vi "Processing_Tracks_Without_Problems-7.vi"(5 "[IN] Min TRK L":i32, 6 "[IN] Max angle between \ntwo displacements":dbl min=1.0 max=90.0 step=1.0, 7 "[IN] % linearity":i32, 8 "error IN":errorcluster, 9 "[IN] Movie Values":T2 {"Particle Fil Setups"."Type of particle filter"."Measurement Parameter" items=["Center of Mass X", "Center of Mass Y", "First Pixel X", "First Pixel Y", "Bounding Rect Left", "Bounding Rect Top", "Bounding Rect Right", "Bounding Rect Bottom", "Max Feret Diameter Start X", "Max Feret Diameter Start Y", "Max Feret Diameter End X", "Max Feret Diameter End Y", "Max Horiz. Segment Length Left", "Max Horiz. Segment Length Right", "Max Horiz. Segment Length Row", "-", "Bounding Rect Width", "Bounding Rect Height", "Bounding Rect Diagonal", "Perimeter", "Convex Hull Perimeter", "Holes' Perimeter", "Max Feret Diameter", "Equivalent Ellipse Major Axis", "Equivalent Ellipse Minor Axis", "Equivalent Ellipse Minor Axis (Feret)", "Equivalent Rect Long Side", "Equivalent Rect Short Side", "Equivalent Rect Diagonal", "Equivalent Rect Short Side (Feret)", "Average Horiz. Segment Length", "Average Vert. Segment Length", "Hydraulic Radius", "Waddel Disk Diameter", "-", "Area", "Holes' Area", "Particle & Holes' Area", "Convex Hull Area", "Image Area", "-", "Number of Holes", "Number of Horiz. Segments", "Number of Vert. Segments", "-", "Orientation", "Max Feret Diameter Orientation", "-", "% Area/Image Area", "% Area/(Particle & Holes' Area)", "Ratio of Equivalent Ellipse Axes", "Ratio of Equivalent Rect Sides", "-", "Elongation Factor", "Compactness Factor", "Heywood Circularity Factor", "Type Factor", "-", "Sum X", "Sum Y", "Sum XX", "Sum XY", "Sum YY", "Sum XXX", "Sum XXY", "Sum XYY", "Sum YYY", "-", "Moment of Inertia XX", "Moment of Inertia XY", "Moment of Inertia YY", "Moment of Inertia XXX", "Moment of Inertia XXY", "Moment of Inertia XYY", "Moment of Inertia YYY", "Norm. Moment of Inertia XX", "Norm. Moment of Inertia XY", "Norm. Moment of Inertia YY", "Norm. Moment of Inertia XXX", "Norm. Moment of Inertia XXY", "Norm. Moment of Inertia XYY", "Norm. Moment of Inertia YYY", "Hu Moment 1", "Hu Moment 2", "Hu Moment 3", "Hu Moment 4", "Hu Moment 5", "Hu Moment 6", "Hu Moment 7"]}, 11 "[IN] Tracks w/t Problems":T3(array[cluster])) -> (0 "error OUT":errorcluster, 2 "[OUT] Filtered Tracks":T3(array[cluster]), 3 "[OUT] Frame-to-Frame Displacements\n Extract From Tracks":dbl[][](array[numeric]))   [LabVIEW 2013]
doc: "SubVI processes the track depending on few parameters: linearity (processivity), length, area differences between connected particles (utilized the properties of the distribution of these differences)"
panel:
  out "[OUT] Filtered out\nShort Tracks":cluster{"Short Tracks":dbl[], "Start Pos":i32}[](array[cluster])
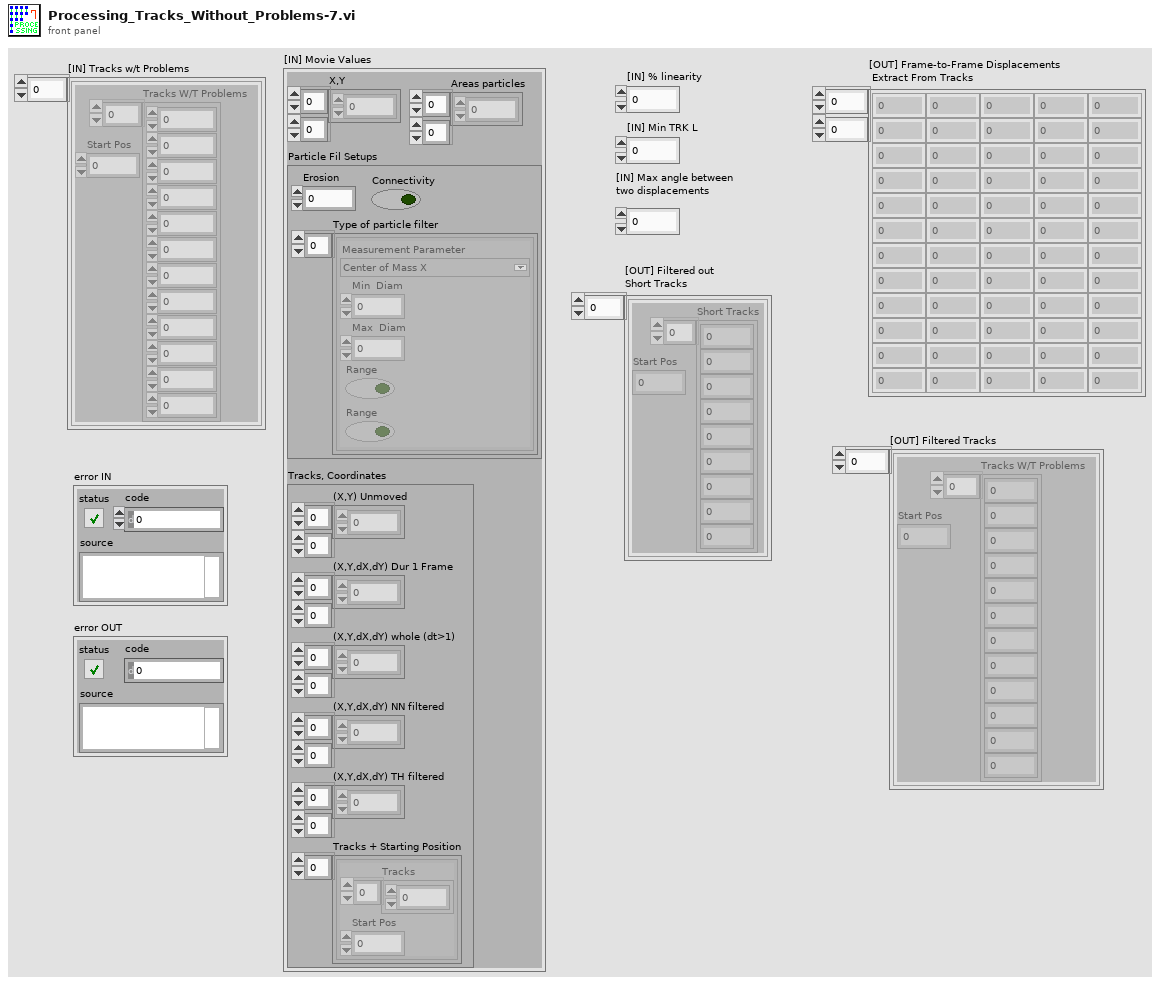
[diagram p1: front panel]
types:
  T1 = typedef "Particle Parameters" = i32
  T2 = cluster{"X,Y":dbl[][], "Areas particles":dbl[][], "Particle Fil Setups":cluster{"Erosion":i32, "Connectivity ":bool, "Type of particle filter":cluster{"Measurement Parameter":T1, "Min  Diam":dbl, "Max  Diam":dbl, "Range":bool, "Range":bool}[]}, "Tracks, Coordinates":cluster{"(X,Y) Unmoved":dbl[][], "(X,Y,dX,dY) Dur 1 Frame":dbl[][], "(X,Y,dX,dY) whole (dt>1)":dbl[][], "(X,Y,dX,dY) NN filtered":dbl[][], "(X,Y,dX,dY) TH filtered":dbl[][], "Tracks + Starting Position":cluster{"Tracks":dbl[], "Start Pos":i32}[]}}
  T3 = cluster{"Tracks W/T Problems":dbl[], "Start Pos":i32}[]
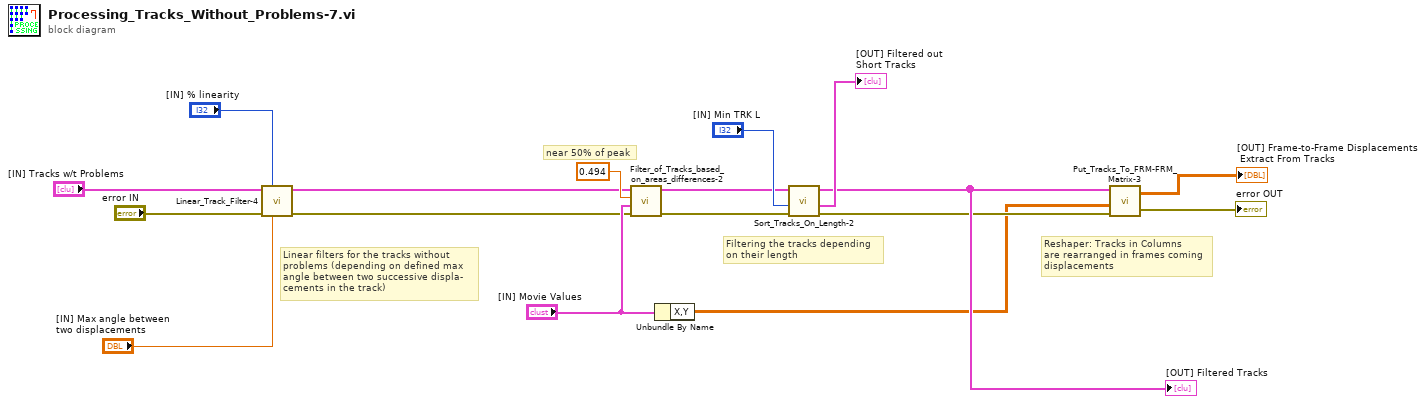
[diagram p0: block diagram]
diagram:
  # "near 50% of peak"
  # "Filtering the tracks depending\non their length"
  # "Linear filters for the tracks without \nproblems (depending on defined max\nangle between two successive displa-\ncements in the track)"
  # "Reshaper: Tracks in Columns\nare rearranged in frames coming\ndisplacements"
  n1 = call "Linear_Track_Filter-4.vi"("[IN] Max angle"="[IN] Max angle between \ntwo displacements", "[IN] % track linearity"="[IN] % linearity", "error IN"="error IN", "[IN] Tracks w/t Problems"="[IN] Tracks w/t Problems") -> ("error OUT"=w2:errorcluster, "[OUT] Linear Tracks (Filtered)"=w4:T3)  [unwired: 5 in, 1 out]
  n2 = call "Filter_of_Tracks_based_on_areas_differences-2.vi"("error IN"=w2, "[IN] Movie Values"="[IN] Movie Values", "[IN] Part of mean value (amplitude)\nFor making filtering criteria"=0.494 ("[IN] Part of mean value (amplitude)\nFor making filtering criteria"), "[IN] Tracks w/t Problems"=w4) -> ("error OUT"=w9:errorcluster, "[OUT] Stable Tracks (Filtered)"=w10:T3)  [unwired: 1 in, 1 out]
  n3 = Unbundle By Name("[IN] Movie Values") -> ("X,Y"=w7:dbl[][])
  n4 = call "Sort_Tracks_On_Length-2.vi"("error IN"=w9, "[IN] Min Track Length"="[IN] Min TRK L", "[IN] Tracks w/t Problems"=w10) -> ("error OUT"=w12:errorcluster, "[OUT] Short Tracks"=→"[OUT] Filtered out\nShort Tracks":cluster{"Short Tracks":dbl[], "Start Pos":i32}[], "[OUT] Long Tracks (Filtered)"=w13:T3)  [unwired: 2 in]
  "[OUT] Filtered Tracks" <- w13
  n5 = call "Put_Tracks_To_FRM-FRM_Matrix-3.vi"("error IN"=w12, "[IN] Matrix for Estimation \nSizes of Frame-to-Frame \nDisplacements from Tracks"=w7, "[IN] Tracks w/t Problems"=w13) -> ("error OUT"=→"error OUT":errorcluster, "[OUT] Frame-to-Frame\nDisplacements Extract\nFrom Tracks"=→"[OUT] Frame-to-Frame Displacements\n Extract From Tracks":dbl[][])  [unwired: 1 in]
